vi "tcs_putSample_WEP.vi"(8 "error in (no error)":errorcluster, 11 "WEP_Ctl":T1) -> (0 "error out":errorcluster, 2 "function return":i32, 3 "WEP_Ctl out":T1)   [LabVIEW 2016, in "SALLV_tcs.lvlib"]
doc: "int tcs_shm_putSample_WEPLV(tcs_WEPLV *WEP_Ctl );"
uses:
  SALLV_tcs.lvlib
  DataTypes/WEP.ctl
  SALLV_tcs.so
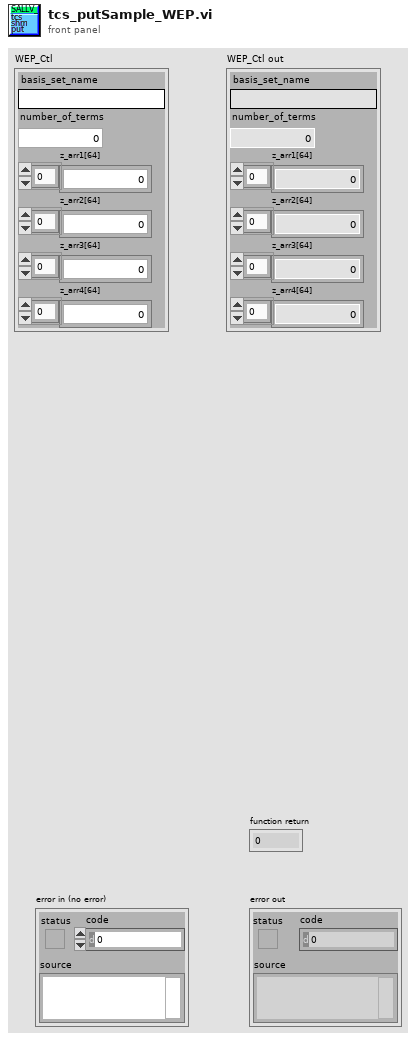
[diagram p1: front panel]
types:
  T1 = typedef "SALLV_tcs.lvlib/WEP.ctl" = cluster{"basis_set_name":string, "number_of_terms":i32, "z_arr1[64]":dbl[], "z_arr2[64]":dbl[], "z_arr3[64]":dbl[], "z_arr4[64]":dbl[]}
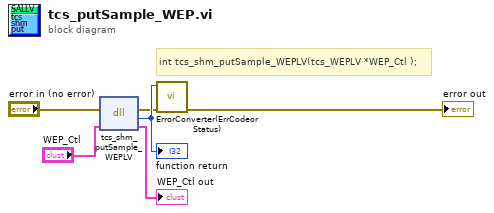
[diagram p0: block diagram]
diagram:
  # "int tcs_shm_putSample_WEPLV(tcs_WEPLV *WEP_Ctl );"
  n1 = dll-call lib="home/andres/Desktop/SALLV_tcs/SALLV_tcs.*" fn="tcs_shm_putSample_WEPLV"(error in="error in (no error)", "WEP_Ctl"="WEP_Ctl") -> (error out=w2:errorcluster, w6:i32, "WEP_Ctl"=→"WEP_Ctl out":T1)  [unwired: 2 in, 1 out]
  "function return" <- w6
  n2 = call "ErrorConverter(ErrCodeorStatus).vi"("error in (no error)"=w2, "error code"=w6) -> ("error out"=→"error out":errorcluster)  [unwired: 9 in]
